vi "绘制图形.vi"(8 "error in (no error)":errorcluster caption="错误输入（无错误）", 10 "Picture in":picture caption="图片输入", 11 "图形 输入":refnum<class "图形.lvclass"> caption="DNL_LabVIEW Object in") -> (0 "error out":errorcluster caption="错误输出", 2 "Picture out":picture caption="图片输出", 3 "图形 输出":refnum<class "图形.lvclass"> caption="DNL_LabVIEW Object out")   [LabVIEW 2011, in "图形.lvclass"]
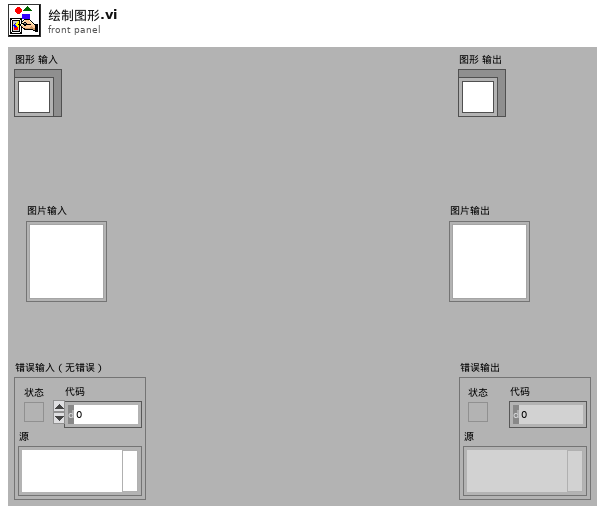
[diagram p1: front panel]
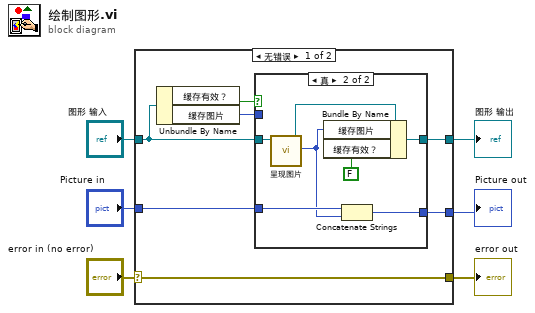
[diagram p0: block diagram]
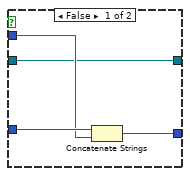
[diagram p2: hidden frame]
diagram:
  n1 = case shown="无错误" "error in (no error)" {
    selector: "error in (no error)" -> [w13 w27]
    tunnel: [w13 w27] -> w5
    tunnel: [w8 w26] -> w3
    tunnel: "图形 输入" -> [w11 w26]
    tunnel: "Picture in" -> [w10 w25]
    tunnel: [w9 w25] -> w1
    frame No Error {
      n2 = Unbundle By Name(w11) -> ("缓存有效？"=w12:bool, "缓存图片"=w7:picture)
      n3 = case shown="真" w12 {
        tunnel: w11 -> [w14 w24]
        tunnel: w10 -> [w17 w23]
        tunnel: [w15 w22] -> w9
        tunnel: [w14 w19] -> w8
        tunnel: w7 -> [w16 _]
        frame False {
          n4 = Concatenate Strings(w17, w16) -> (w15:picture)
        }
        frame True {
          n5 = call-dynamic "呈现图片.vi"("图形 输入"=w24) -> ("Picture"=w18:picture, "图形 输出"=w21:refnum<class "图形.lvclass">)  [unwired: 8 in, 1 out]
          n6 = Bundle By Name(cluster=w21, "缓存图片"=w18, "缓存有效？"=FALSE) -> (w19:refnum<class "图形.lvclass">)
          n7 = Concatenate Strings(w23, w18) -> (w22:picture)
        }
      }
    }
    frame Error {
    }
  }
  "error out" <- w5
  "图形 输出" <- w3
  "Picture out" <- w1
